vi "L1.vi"() -> ()   [LabVIEW 2014]
panel:
  out "Radacini reale":bool
  out "DELTA":dbl
  out "X2":dbl format="%#_3g"
  out "X1":dbl format="%#_3g"
  in  "C":dbl(slide) scale=-10.0..10.0
  in  "B":dbl(slide) scale=-10.0..10.0
  in  "A":dbl(slide) scale=-10.0..10.0
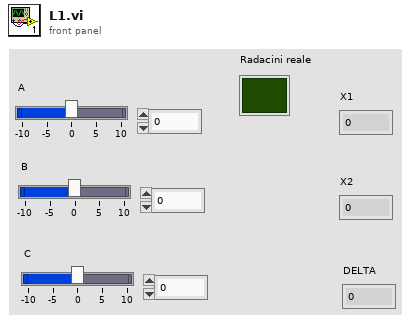
[diagram p1: front panel]
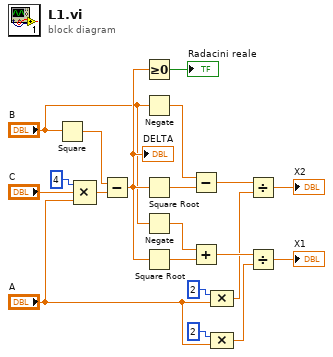
[diagram p0: block diagram]
diagram:
  n1 = Square(x="B") -> (x^2=w20:dbl)
  n2 = Compound Arithmetic op=MULTIPLY(4, "C", "A") -> (w17:dbl)
  n3 = Subtract(x=w20, y=w17) -> (x-y=w4:dbl)
  "DELTA" <- w4
  n4 = Greater Or Equal To 0?(x=w4) -> (x >= 0?=→"Radacini reale":bool)
  n5 = Negate(x="B") -> (-x=w9:dbl)
  n6 = Square Root(x=w4) -> (sqrt(x)=w8:dbl)
  n7 = Negate(x="B") -> (-x=w15:dbl)
  n8 = Square Root(x=w4) -> (sqrt(x)=w14:dbl)
  n9 = Subtract(x=w9, y=w8) -> (x-y=w5:dbl)
  n10 = Add(x=w15, y=w14) -> (x+y=w11:dbl)
  n11 = Compound Arithmetic op=MULTIPLY(2, "A") -> (w6:dbl)
  n12 = Compound Arithmetic op=MULTIPLY(2, "A") -> (w12:dbl)
  n13 = Divide(x=w5, y=w6) -> (x/y=→"X2":dbl)
  n14 = Divide(x=w11, y=w12) -> (x/y=→"X1":dbl)
